vi "Teleop.vi"(10 "Match Info":T1={"Autonomous Elapsed Seconds"=0.0, "TeleOp Elapsed Seconds"=0.0, "Disabled Elapsed Seconds"=0.0, "Visited Autonomous"=FALSE, "Visited TeleOp"=FALSE, "Visited Disabled"=FALSE, "Autonomous Settings"={"Autonomous Style"=enum."Independent", "VI Refnum"=refnum}}, 11 "Call Context":T2) -> ()   [LabVIEW 2016]
doc: "This VI is called for each TeleOp packet received from the DS where the robot is not disabled. It is often used to read from the joysticks and update I/O or to update setpoints for timed control loops. It should complete and return within 20 milliseconds or it may miss DS packets."
uses:
  <vilib>/Rock Robotics/WPI/DriverStation/WPI_DriverStationDerivedRobotMode.ctl
  <vilib>/Rock Robotics/WPI/DriverStation/WPI_DriverStationMatch Info.ctl
  <vilib>/Rock Robotics/WPI/Utilities/WPI_GetSetVariantRefNum.vi
  <vilib>/Rock Robotics/Network Tables/NT Write Boolean Array.vi
  <vilib>/Rock Robotics/Network Tables/NT Write Numeric Array.vi
  <vilib>/Rock Robotics/Network Tables/NT Read Boolean.vi
  <vilib>/Rock Robotics/Network Tables/NT Read Number.vi
  <vilib>/Rock Robotics/Network Tables/NT Write Number.vi
  <vilib>/Rock Robotics/WPI/RobotDrive/WPI_RobotDriveMecanumDrive_Cartesian.vi
  ADIS16448-RoboRIO-Driver/LabVIEW/ADI MXP IMU/FRC_ADIS16448_IMU.lvlib
panel:
  out "Sample Slider 0":dbl(slide) scale=0.0..5.0
  out "Sample Boolean 1":bool
  out "Sample Boolean 0":bool
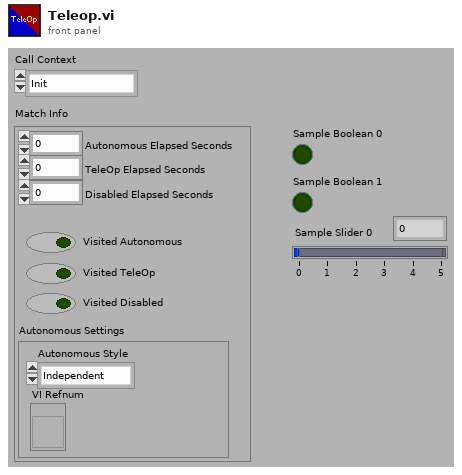
[diagram p1: front panel]
types:
  T1 = typedef "WPI_DriverStationMatch Info.ctl" = cluster{"Autonomous Elapsed Seconds":dbl, "TeleOp Elapsed Seconds":dbl, "Disabled Elapsed Seconds":dbl, "Visited Autonomous":bool, "Visited TeleOp":bool, "Visited Disabled":bool, "Autonomous Settings":cluster{"Autonomous Style":enum16{"Iterative", "Independent"}, "VI Refnum":refnum<vi>}}
  T2 = typedef "WPI_DriverStationDerivedRobotMode.ctl" = enum16{"Init", "Execute", "Stop"}
  T3 = typedef "WPI_RobotDriveDevRef.ctl" = cluster{"DevStatus":errorcluster, "Motors[]":T4[], "Square Inputs":bool, "Max Output":dbl}
  T4 = typedef "WPI_MotorControlDeviceRef.ctl" = cluster{"DeviceStatus":errorcluster, "Type":T5, "PWM":cluster{"PWM Channel":T6, "DeadBand":T7}, "CAN":cluster{"Device Number":u8, "SetOutput VI Ref":variant, "GetOutput VI Ref":variant, "Enable VI Ref":variant, "Disable VI Ref":variant, "Data":variant}, "Invert":bool}
  T5 = typedef "WPI_MotorControlType.ctl" = enum16{"PWM", "CAN"}
  T6 = typedef "FPGA_DIOPWMChannel.ctl" = enum8{"PWM 0", "PWM 1", "PWM 2", "PWM 3", "PWM 4", "PWM 5", "PWM 6", "PWM 7", "PWM 8", "PWM 9", "PWM MXP 0", "PWM MXP 1", "PWM MXP 2", "PWM MXP 3", "PWM MXP 4", "PWM MXP 5", "PWM MXP 6", "PWM MXP 7", "PWM MXP 8", "PWM MXP 9", "Invalid"}
  T7 = typedef "WPI_PWMDeadband.ctl" = cluster{"Name":string, "maxPositivePwm":i32, "minPositivePwm":i32, "centerPwm":i32, "maxNegativePwm":i32, "minNegativePwm":i32, "angularRange":u16}
  T8 = typedef "WPI_JoystickDevRef.ctl" = cluster{"Device":T9}
  T9 = typedef "WPI_JoystickDeviceEnum.ctl" = enum16{"USB 0", "USB 1", "USB 2", "USB 3", "USB 4", "USB 5"}
  T10 = typedef "FRC_ADIS16448_IMU.lvlib/WPI_IMU_ADIS16448_InterruptDevRef.ctl" = cluster{"ADI IMU DevRef":T11, "InterruptRef":T13}
  T11 = typedef "FRC_ADIS16448_IMU.lvlib/WPI_IMU_ADIS16448_IMUDevRef.ctl" = cluster{"DevStatus":errorcluster, "Handle":i32, "SPI Bus":T12, "Device Found":bool, "Device Ready":bool, "Yaw Axis":enum16{"X", "Y", "Z"}, "AHRS Algorithm":enum16{"Complementary", "Madgwick"}, "Serial":u16, "Lot ID 2":u16, "Lot ID 1":u16, "Product ID":u16}
  T12 = typedef "spi_bus.ctl" = enum16{"SPI On-Board, CS0", "SPI On-Board, CS1", "SPI On-Board, CS2", "SPI On-Board, CS3", "SPI MXP", "Invalid"}
  T13 = typedef "WPI_InterruptRef.ctl" = cluster{"DevStatus":errorcluster, "InterruptIndex":T14}
  T14 = typedef "FPGA_InterruptIndex.ctl" = enum8{"0", "1", "2", "3", "4", "5", "6", "7", "Invalid"}
  T15 = cluster{"X Angle":dbl, "Y Angle":dbl, "Z Angle":dbl}
  T16 = typedef "WPI_ServoDeviceRef.ctl" = cluster{"DeviceStatus":errorcluster, "PWM Channel":T6, "DeadBand":T7}
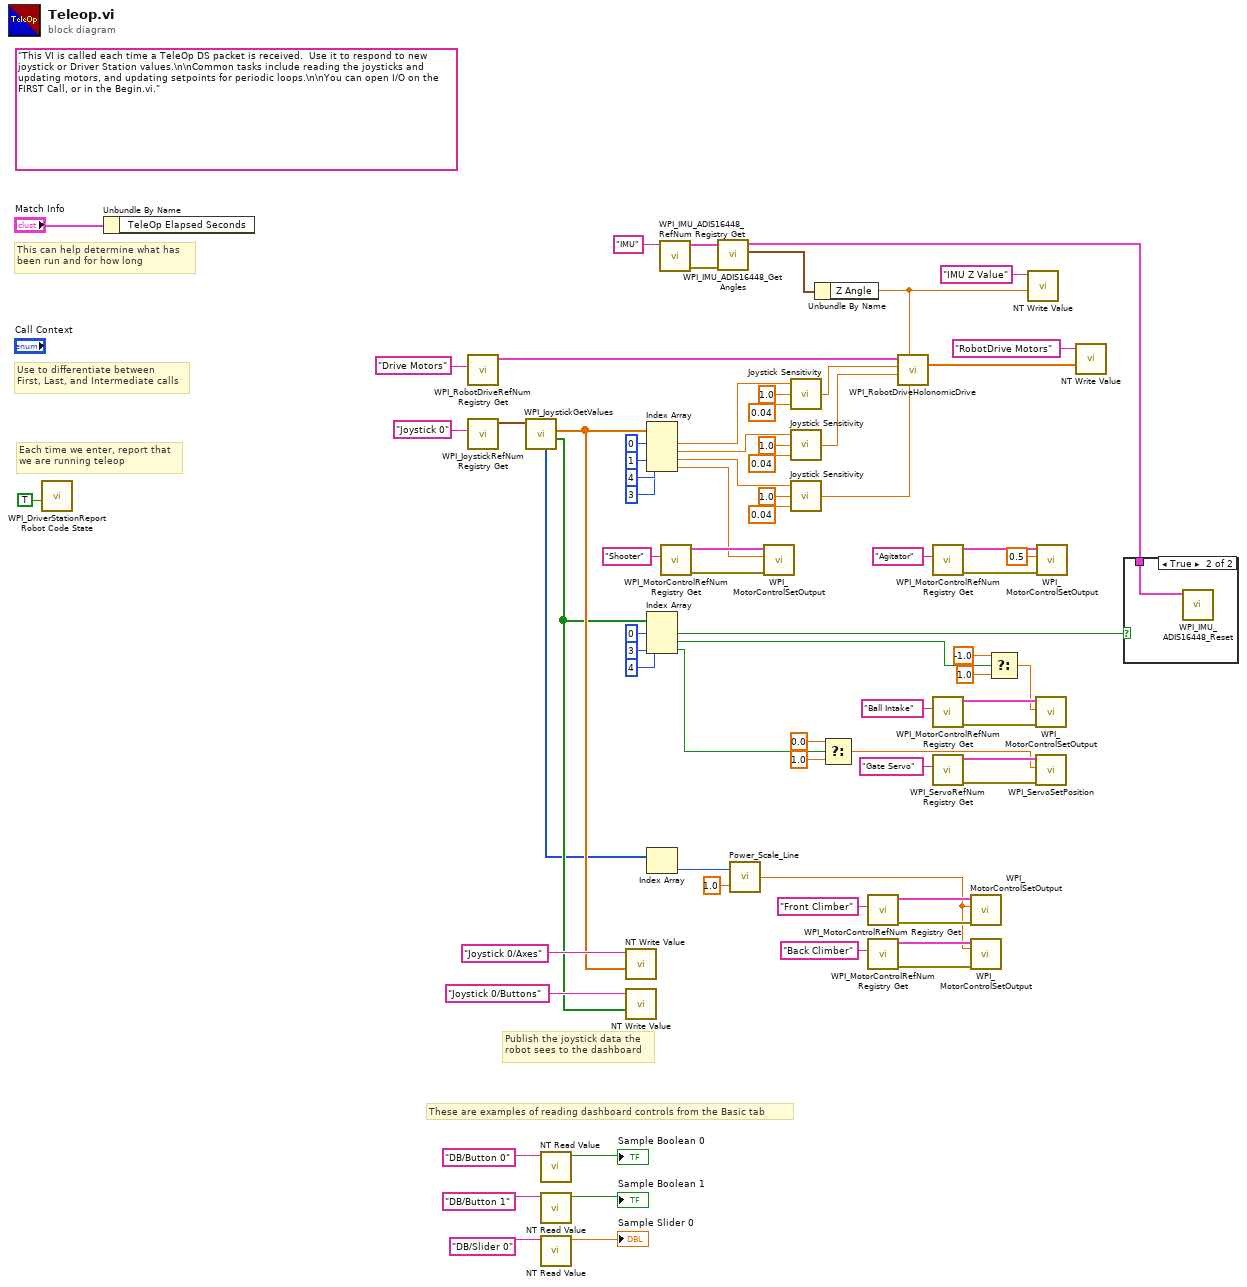
[diagram p0: block diagram]
diagram:
  (unwired) "This VI is called each time a TeleOp DS packet is received.  Use it to respond to new joystick or Driver Station values.\n\nCommon tasks include reading the joysticks and updating motors, and updating setpoints for periodic loops.\n\nYou can open I/O on the FIRST Call, or in the Begin.vi."
  # "These are examples of reading dashboard controls from the Basic tab"
  # "Publish the joystick data the\nrobot sees to the dashboard"
  # "Each time we enter, report that\nwe are running teleop"
  # "Use to differentiate between\nFirst, Last, and Intermediate calls"
  # "This can help determine what has\nbeen run and for how long"
  n1 = call <vilib>:"WPI_DriverStationReport Robot Code State.vi"("TeleOp"=TRUE ("Autonomous")) -> ()  [unwired: 10 in, 1 out]
  n2 = Unbundle By Name("Match Info") -> ()  [unwired: 1 out]
  n3 = call <vilib>:"WPI_RobotDriveRefNum Registry Get.vi"("refnum name"="Drive Motors") -> ("RobotDriveDevRef"=w75:T3)  [unwired: 1 in, 9 out]
  n4 = call <vilib>:"WPI_JoystickRefNum Registry Get.vi"("refnum name"="Joystick 0") -> ("JoystickDevRef"=w73:T8)  [unwired: 1 in, 9 out]
  n5 = call <vilib>:"WPI_JoystickGetValues.vi"("JoystickDevRef"=w73) -> ("Buttons"=w44:bool[], "Axes"=w70:dbl[], "POVs"=w16:i16[])  [unwired: 6 in, 2 out]
  n6 = call-poly <vilib>:"NT Read Value.vi"("Name"="DB/Button 0" ("refnum name")) -> ("Boolean"=→"Sample Boolean 0":bool)  [unwired: 9 in, 1 out]
  n7 = call-poly <vilib>:"NT Read Value.vi"("Name"="DB/Button 1" ("refnum name")) -> ("Boolean"=→"Sample Boolean 1":bool)  [unwired: 9 in, 1 out]
  n8 = call-poly <vilib>:"NT Read Value.vi"("Name"="DB/Slider 0" ("refnum name")) -> ("Numeric"=→"Sample Slider 0":dbl)  [unwired: 9 in, 1 out]
  n9 = call-poly <vilib>:"NT Write Value.vi"("Numeric Array"=w70, "Name"="Joystick 0/Axes") -> ()  [unwired: 9 in, 1 out]
  n10 = call-poly <vilib>:"NT Write Value.vi"("Boolean Array"=w44, "Name"="Joystick 0/Buttons") -> ()  [unwired: 9 in, 1 out]
  n11 = Index Array(array=w70, index #1=0 ("index"), index #2=1 ("index"), index #3=4 ("index"), index #4=3 ("index")) -> (element #1=w50:dbl, element #2=w53:dbl, element #3=w54:dbl, element #4=w31:dbl)
  n12 = Index Array(array=w44, index #1=0 ("index"), index #2=3 ("index"), index #3=4 ("index")) -> (element #1=w42:bool, element #2=w22:bool, element #3=w4:bool)
  n13 = Index Array(array=w16) -> (element=w18:i16)  [unwired: 1 in]
  n14 = call "WPI_IMU_ADIS16448_RefNum Registry Get.vi"("refnum name"="IMU") -> ("error out"=w40:errorcluster, "ADI IMU Interrupt DevRef"=w41:T10)  [unwired: 9 in]
  n15 = call <vilib>:"WPI_MotorControlRefNum Registry Get.vi"("refnum name"="Shooter") -> ("error out"=w34:errorcluster, "MotorControlDevRef"=w35:T4)  [unwired: 9 in]
  n16 = call "WPI_IMU_ADIS16448_Get Angles.vi"("error in"=w40, "ADI IMU Interrupt DevRef"=w41) -> ("IMU Angles Out"=w36:T15, "ADI IMU Interrupt DevRef Out"=w39:T10)  [unwired: 6 in, 2 out]
  n17 = call "Power_Scale_Line.vi"("Power Input"=1.0, "POV"=w18) -> ("Power Output"=w9:dbl)
  n18 = call <vilib>:"WPI_MotorControlSetOutput.vi"("error in (no error)"=w34, "Output"=w31, "MotorControlDevRef"=w35) -> ()  [unwired: 6 in, 3 out]
  n19 = call "Joystick Sensitivity.vi"("B"=0.04, "A"=1.0, "X"=w50) -> ("Y"=w47:dbl)
  n20 = call "Joystick Sensitivity.vi"("B"=0.04, "A"=1.0, "X"=w53) -> ("Y"=w46:dbl)
  n21 = call "Joystick Sensitivity.vi"("B"=0.04, "A"=1.0, "X"=w54) -> ("Y"=w57:dbl)
  n22 = Unbundle By Name(w36) -> ("Z Angle"=w37:dbl)
  n23 = Select(t=0.0, s=w4, f=1.0) -> (s? t:f=w1:dbl)
  n24 = call <vilib>:"WPI_MotorControlRefNum Registry Get.vi"("refnum name"="Front Climber") -> ("error out"=w14:errorcluster, "MotorControlDevRef"=w15:T4)  [unwired: 9 in]
  n25 = call <vilib>:"WPI_MotorControlRefNum Registry Get.vi"("refnum name"="Back Climber") -> ("error out"=w11:errorcluster, "MotorControlDevRef"=w12:T4)  [unwired: 9 in]
  n26 = call-poly <vilib>:"WPI_RobotDriveHolonomicDrive.vi"("Rotation"=w57, "Gyro Angle"=w37, "Y"=w46, "X"=w47, "RobotDriveDevRef"=w75) -> ("Motor Values"=w68:dbl[])  [unwired: 4 in, 2 out]
  n27 = call <vilib>:"WPI_MotorControlRefNum Registry Get.vi"("refnum name"="Agitator") -> ("error out"=w29:errorcluster, "MotorControlDevRef"=w30:T4)  [unwired: 9 in]
  n28 = call <vilib>:"WPI_MotorControlRefNum Registry Get.vi"("refnum name"="Ball Intake") -> ("error out"=w25:errorcluster, "MotorControlDevRef"=w26:T4)  [unwired: 9 in]
  n29 = call <vilib>:"WPI_ServoRefNum Registry Get.vi"("refnum name"="Gate Servo") -> ("error out"=w7:errorcluster, "ServoDeviceRef"=w8:T16)  [unwired: 9 in]
  n30 = call <vilib>:"WPI_MotorControlSetOutput.vi"("error in (no error)"=w14, "Output"=w9, "MotorControlDevRef"=w15) -> ()  [unwired: 6 in, 3 out]
  n31 = call <vilib>:"WPI_MotorControlSetOutput.vi"("error in (no error)"=w11, "Output"=w9, "MotorControlDevRef"=w12) -> ()  [unwired: 6 in, 3 out]
  n32 = Select(t=-1.0, s=w22, f=1.0) -> (s? t:f=w24:dbl)
  n33 = call-poly <vilib>:"NT Write Value.vi"("Numeric"=w37, "Name"="IMU Z Value") -> ()  [unwired: 9 in, 1 out]
  n34 = call <vilib>:"WPI_MotorControlSetOutput.vi"("error in (no error)"=w25, "Output"=w24, "MotorControlDevRef"=w26) -> ()  [unwired: 6 in, 3 out]
  n35 = call <vilib>:"WPI_ServoSetPosition.vi"("error in (no error)"=w7, "Position"=w1, "ServoDeviceRef"=w8) -> ()  [unwired: 7 in, 2 out]
  n36 = call <vilib>:"WPI_MotorControlSetOutput.vi"("error in (no error)"=w29, "Output"=0.5, "MotorControlDevRef"=w30) -> ()  [unwired: 6 in, 3 out]
  n37 = call-poly <vilib>:"NT Write Value.vi"("Numeric Array"=w68, "Name"="RobotDrive Motors") -> ()  [unwired: 9 in, 1 out]
  n38 = case shown="True" w42 {
    tunnel: w39 -> [_ w78]
    frame False {
    }
    frame True {
      n39 = call "WPI_IMU_ADIS16448_Reset.vi"("ADI IMU Interrupt DevRef"=w78) -> ()  [unwired: 9 in, 2 out]
    }
  }
